vi "Prober_LoadUnload.vi"(8 "error in (no error)":errorcluster, 11 "SemiProbe in":refnum<class "SemiProbe.lvclass">) -> (0 "error out":errorcluster, 2 "Home or Load?":enum16{"Measure", "Load"}(ring), 3 "SemiProbe out":refnum<class "SemiProbe.lvclass">)   [LabVIEW 2019, in "SemiProbe.lvclass"]
uses:
  SemiProbe.lvclass
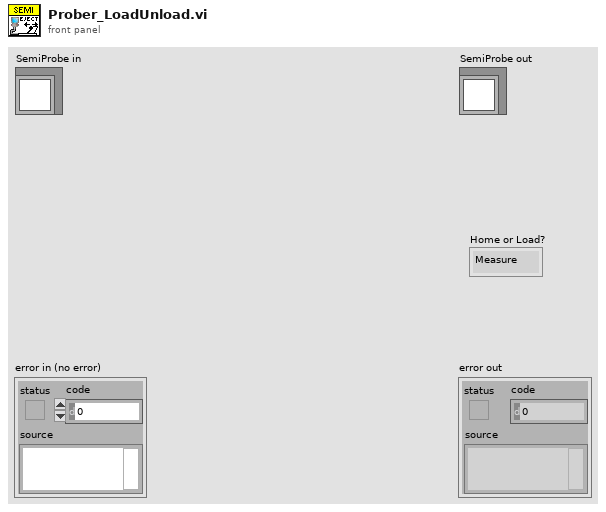
[diagram p1: front panel]
types:
  T1 = enum16{"Move To Load", "Move To Double Separation", "Move To Separation Distance", "Move To Contact", "Execute Contact Search", "Execute Arduino Contact Search"}
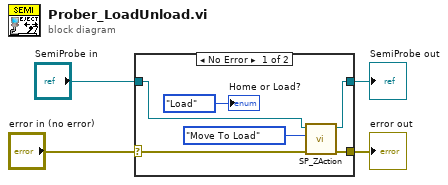
[diagram p0: block diagram]
diagram:
  n1 = case shown="No Error" "error in (no error)" {
    selector: "error in (no error)" -> [w8 w11]
    tunnel: "SemiProbe in" -> [w9 w12]
    tunnel: [w6 w12] -> w2
    tunnel: [w7 w11] -> w1
    frame No Error {
      n2 = call-dynamic "SP_ZAction.vi"("error in (no error)"=w8, "Z Action"=T1."Move To Load", "SemiProbe in"=w9) -> ("error out"=w7:errorcluster, "SemiProbe out"=w6:refnum<class "SemiProbe.lvclass">)  [unwired: 5 in, 2 out]
      "Home or Load?" <- enum16{"Measure", "Load"}."Load" ("Home or Load?")
    }
    frame Error {
    }
  }
  "error out" <- w1
  "SemiProbe out" <- w2
